vi "ServiceMonitor.vi"(1 "STOP":bool) -> (0 "Stop?":bool)   [LabVIEW 2011]
panel:
  # "This VI called via VI server\nfrom EndService.vi (built into\nserver.dll).  Don't change it's\nconnector pane without checking\nin that location."
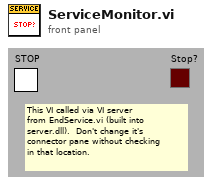
[diagram p1: front panel]
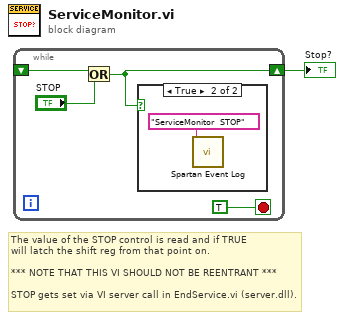
[diagram p0: block diagram]
diagram:
  # "The value of the STOP control is read and if TRUE\nwill latch the shift reg from that point on.\n\n*** NOTE THAT THIS VI SHOULD NOT BE REENTRANT ***\n\nSTOP gets set via VI server call in EndService.vi (server.dll)."
  n1 = while {
    shift-right: [w2] -> w1
    shift-left: _ -> [w5]
    stop <- TRUE stop-if-true
    n2 = Or(x=w5, y="STOP") -> (x .or. y?=w2:bool)
    n3 = case shown="True" w2 {
      frame False {
      }
      frame True {
        n4 = call "Spartan Event Log.vi"("message (\"\")"="ServiceMonitor  STOP") -> ()  [unwired: 4 in, 4 out]
      }
    }
  }
  "Stop?" <- w1
